vi "4155C Config Sampling Measurements v2.0.vi"(0 "VISA session":refnum<visa-resource-name>, 1 "Num Points":i16=1 min=1 max=1001, 2 "Sample - Drain":u32(ring)=1 items=["SMU1  ", "SMU2  ", "SMU3  ", "SMU4  ", "SMU5  ", "SMU6  "], 3 "Display on/off":bool, 5 "Gate Compliance":dbl format="%.2f", 6 "Sampling interval":dbl min=0.0 max=100000000000.0 format="%.6f", 7 "Sample - Source/Common":u32(ring) items=["SMU1  ", "SMU2  ", "SMU3  ", "SMU4  ", "SMU5  ", "SMU6  "], 8 "Sample - Probe 4":u32(ring)=3 items=["SMU1  ", "SMU2  ", "SMU3  ", "SMU4  ", "SMU5  ", "SMU6  "], 9 "Drain Compliance":dbl format="%.2f", 10 "Standby":T1, 11 "error in (no error)":errorcluster, 12 "Timings":T2={"integration time"=0, "Short/Long integration time"=0.00064, "hold time (sec)"=0.0, "delay time (sec)"=0.0, "Step Time (0 disables)"=0.0, "sweep method"=0, "Pulse period"=0.005, "Base voltage"=0.0, "Pulse width"=0.0005} {"Pulse width" min=0.0005 max=0.1 step=0.0001 format="%.4f"; "Base voltage" min=-100.0 max=100.0 format="%^.4e"; "Pulse period" min=0.005 max=1.0 step=0.0001 format="%.4f"; "sweep method" items=["Continuous", "Pulsed"]; "Step Time (0 disables)" format="%.2f"; "delay time (sec)" min=0.0 format="%.4f"; "hold time (sec)" min=0.0 format="%.4f"; "Short/Long integration time" min=0.0 format="%^.0e"; "integration time" scale=0.0..2.0}, 13 "Sample - Gate":u32(ring)=2 items=["SMU1  ", "SMU2  ", "SMU3  ", "SMU4  ", "SMU5  ", "SMU6  "], 14 "Sample time":dbl min=0.0 max=100000000000.0 format="%.2f") -> (4 "dup VISA resource name":refnum<visa-resource-name>, 15 "error out":errorcluster)   [LabVIEW 2016]
doc: "This VI configures the primary sweep source (VAR1) for a sweep mode measurement. \n* This VI does not perform error checking on MEASUREMENT MODE or UNIT TYPE of VAR1, therefore it is the application programmer's responsibility to make certain this VI is used in the proper mode."
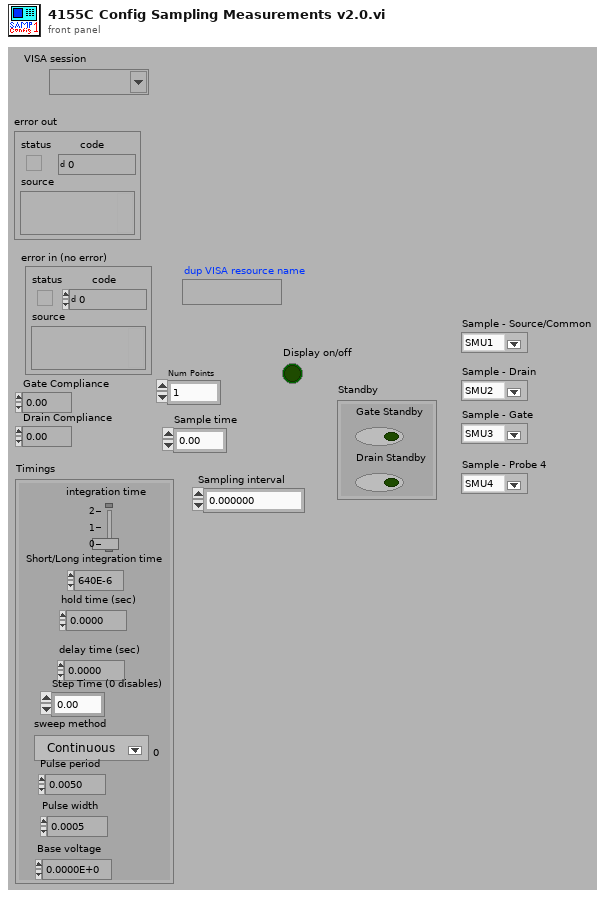
[diagram p1: front panel]
types:
  T1 = cluster{"Gate Standby":bool, "Drain Standby":bool}
  T2 = cluster{"integration time":u32, "Short/Long integration time":dbl, "hold time (sec)":dbl, "delay time (sec)":dbl, "Step Time (0 disables)":dbl, "sweep method":u16, "Pulse period":dbl, "Base voltage":dbl, "Pulse width":dbl}
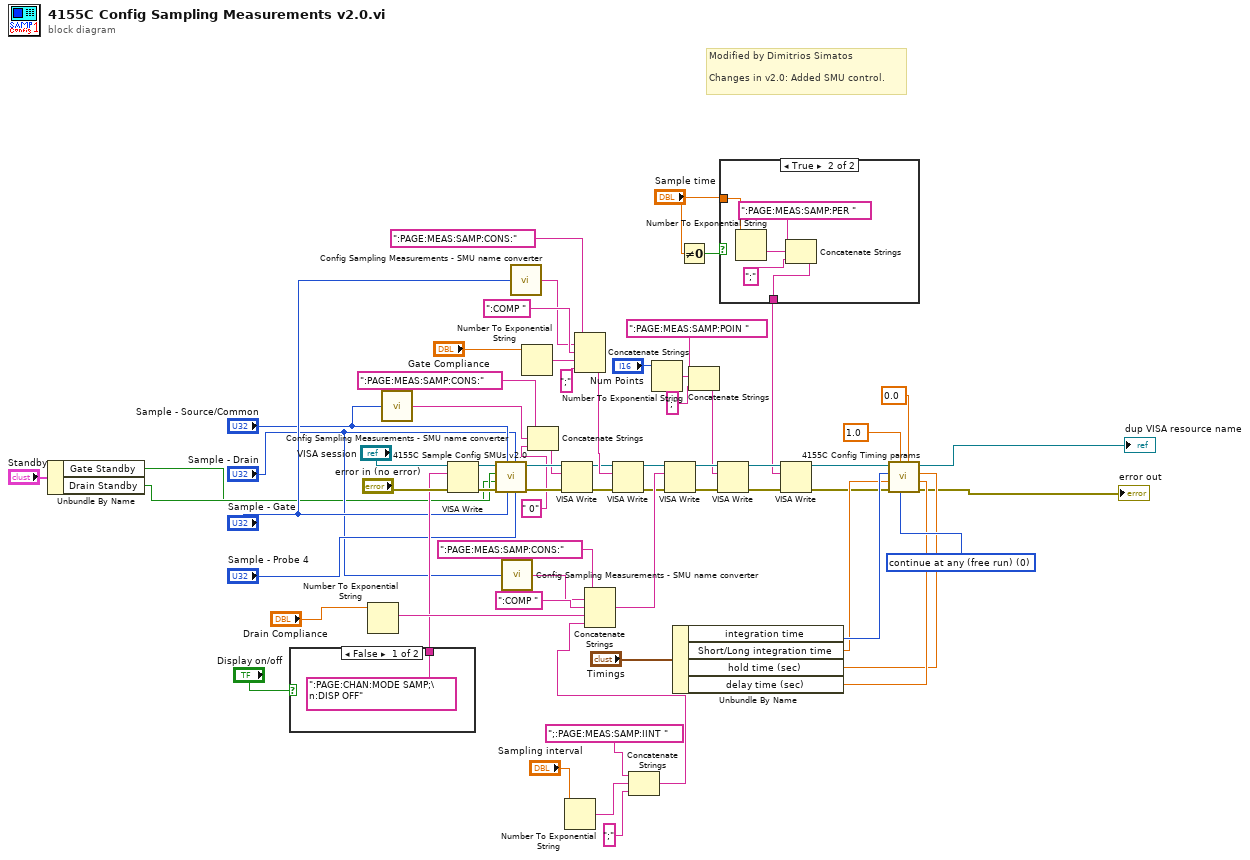
[diagram p0: block diagram]
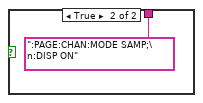
[diagram p2: hidden frame]
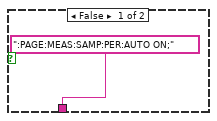
[diagram p3: hidden frame]
diagram:
  w52 = u8 0 items=["continue at any (free run)", "stop at any abnorm", "stop at compliance"] ("stop condition (free run:0)")
  # "Modified by Dimitrios Simatos\n\nChanges in v2.0: Added SMU control."
  n1 = Unbundle By Name("Standby") -> ("Gate Standby"=w1:bool, "Drain Standby"=w2:bool)
  n2 = case shown="False" "Display on/off" {
    tunnel: [":PAGE:CHAN:MODE SAMP;\n:DISP OFF" ("write buffer (\"\")") ":PAGE:CHAN:MODE SAMP;\n:DISP ON" ("write buffer (\"\")")] -> w22
    frame False {
    }
    frame True {
    }
  }
  n3 = Number To Exponential String(number="Drain Compliance") -> (E-format string=w61:string)  [unwired: 3 in]
  n4 = call "Config Sampling Measurements - SMU name converter.vi"("unit to configure"="Sample - Source/Common") -> ("SMU to be configured"=w9:string)
  n5 = VISA Write(VISA resource name="VISA session", write buffer=w22, error in (no error)="error in (no error)") -> (VISA resource name out=w41:refnum<visa-resource-name>, error out=w40:errorcluster)  [unwired: 1 out]
  n6 = call "4155C Sample Config SMUs v2.0.vi"("Sample - Probe 4"="Sample - Probe 4", "Sample - Drain"="Sample - Drain", "Sample - Gate"="Sample - Gate", "Sample - Source/Common"="Sample - Source/Common", "error in (no error)"=w40, "Gate Standby"=w1, "Drain Standby"=w2, "VISA resource name in"=w41) -> ("error out"=w39:errorcluster, "VISA Resource Name out"=w38:refnum<visa-resource-name>)  [unwired: 2 in]
  n7 = call "Config Sampling Measurements - SMU name converter.vi"("unit to configure"="Sample - Drain") -> ("SMU to be configured"=w5:string)
  n8 = call "Config Sampling Measurements - SMU name converter.vi"("unit to configure"="Sample - Gate") -> ("SMU to be configured"=w14:string)
  n9 = Number To Exponential String(number="Gate Compliance") -> (E-format string=w59:string)  [unwired: 3 in]
  n10 = Concatenate Strings(":PAGE:MEAS:SAMP:CONS:" ("write buffer (\"\")"), w9, " 0" ("write buffer (\"\")")) -> (w12:string)
  n11 = VISA Write(VISA resource name=w38, write buffer=w12, error in (no error)=w39) -> (VISA resource name out=w57:refnum<visa-resource-name>, error out=w56:errorcluster)  [unwired: 1 out]
  n12 = Number To Exponential String(number="Sampling interval") -> (E-format string=w21:string)  [unwired: 3 in]
  n13 = Concatenate Strings(":PAGE:MEAS:SAMP:CONS:", w14, ":COMP ", w59, ";" ("Substring")) -> (w60:string)
  n14 = VISA Write(VISA resource name=w57, write buffer=w60, error in (no error)=w56) -> (VISA resource name out=w55:refnum<visa-resource-name>, error out=w54:errorcluster)  [unwired: 1 out]
  n15 = Concatenate Strings(";:PAGE:MEAS:SAMP:IINT ", w21, ";" ("Substring")) -> (w18:string)
  n16 = Concatenate Strings(":PAGE:MEAS:SAMP:CONS:", w5, ":COMP ", w61, w18) -> (w63:string)
  n17 = Number To Exponential String(number="Num Points") -> (E-format string=w36:string)  [unwired: 3 in]
  n18 = VISA Write(VISA resource name=w55, write buffer=w63, error in (no error)=w54) -> (VISA resource name out=w64:refnum<visa-resource-name>, error out=w65:errorcluster)  [unwired: 1 out]
  n19 = Unbundle By Name("Timings") -> ("integration time"=w49:u32, "Short/Long integration time"=w44:dbl, "hold time (sec)"=w50:dbl, "delay time (sec)"=w51:dbl)
  n20 = Not Equal To 0?(x="Sample time") -> (x != 0?=w29:bool)
  n21 = Concatenate Strings(":PAGE:MEAS:SAMP:POIN " ("write buffer (\"\")"), w36, ";" ("Substring")) -> (w31:string)
  n22 = VISA Write(VISA resource name=w64, write buffer=w31, error in (no error)=w65) -> (VISA resource name out=w28:refnum<visa-resource-name>, error out=w27:errorcluster)  [unwired: 1 out]
  n23 = case shown="True" w29 {
    tunnel: "Sample time" -> [_ w72]
    tunnel: [":PAGE:MEAS:SAMP:PER:AUTO ON;" w69] -> w24
    frame False {
    }
    frame True {
      n24 = Number To Exponential String(number=w72) -> (E-format string=w73:string)  [unwired: 3 in]
      n25 = Concatenate Strings(":PAGE:MEAS:SAMP:PER " ("Substring"), w73, ";" ("Substring")) -> (w69:string)
    }
  }
  n26 = VISA Write(VISA resource name=w28, write buffer=w24, error in (no error)=w27) -> (VISA resource name out=w25:refnum<visa-resource-name>, error out=w26:errorcluster)  [unwired: 1 out]
  n27 = call "4155C Config Timing params.vi"("delay time (sec)"=w51, "hold time (sec)"=w50, "Step Time (0 disables)"=0.0, "stop condition (free run:0)"=w52, "wait time parameter"=1.0, "error in (no error)"=w26, "Short/Long integration time"=w44, "integration time"=w49, "VISA session"=w25) -> ("error out"=→"error out":errorcluster, "dup VISA resource name"=→"dup VISA resource name":refnum<visa-resource-name>)  [unwired: 1 in]
